vi "Online_SNR_Add_Measurement.vi"(8 "error in (no error)":errorcluster, 9 "Estimate":dbl format="%#_13g", 10 "True":dbl format="%#_13g", 11 "Online_SNR in":refnum<class "Online_SNR.lvclass">) -> (0 "error out":errorcluster, 3 "Online_SNR out":refnum<class "Online_SNR.lvclass">)   [LabVIEW 2021, in "Online_SNR.lvclass"]
uses:
  Online_SNR.lvclass
  Online_SNR.lvclass/Online_SNR.ctl
  Read Mean Square.vi
  Read Mean Square Error.vi
  Read N.vi
  Write Mean Square.vi
  Write Mean Square Error.vi
  Write N.vi
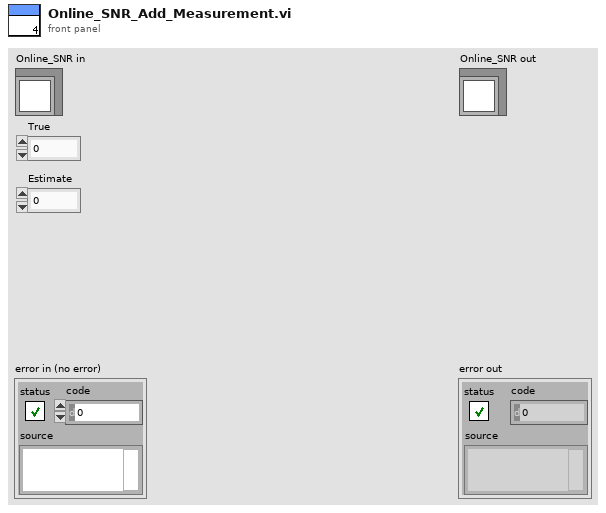
[diagram p1: front panel]
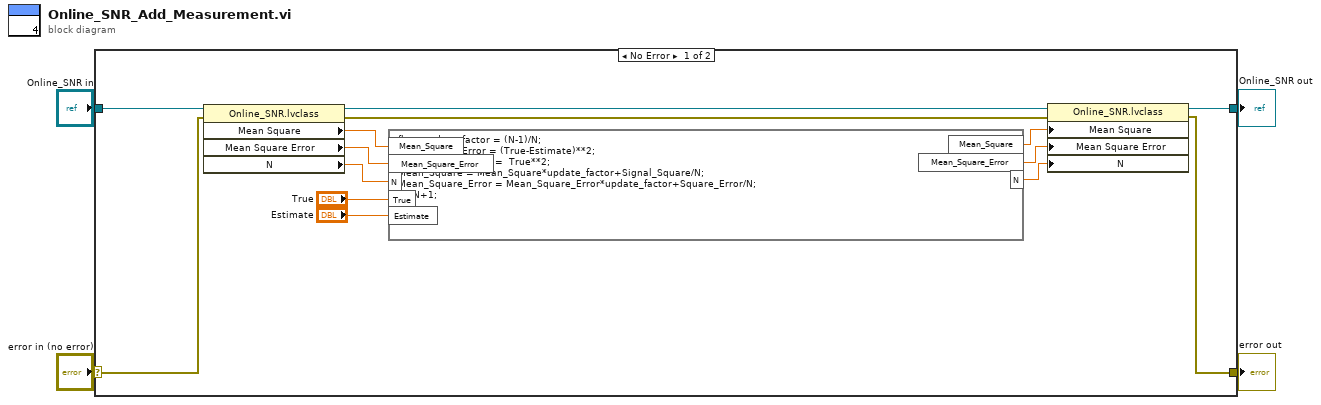
[diagram p0: block diagram]
diagram:
  n1 = case shown="No Error" "error in (no error)" {
    selector: "error in (no error)" -> [w6 w20]
    tunnel: [w5 w20] -> w3
    tunnel: [w9 w19] -> w1
    tunnel: "Online_SNR in" -> [w11 w19]
    frame No Error {
      n2 = property class="Online_SNR.lvclass"(reference=w11, error in=w6) -> (reference out=w10:refnum<class "Online_SNR.lvclass">, error out=w13:errorcluster, "Mean Square"=w18:dbl, "Mean Square Error"=w17:dbl, "N"=w16:dbl)
      n3 = formula code="float update_factor = (N-1)/N;\nfloat Square_Error = (True-Estimate)**2;\nfloat Signal_Square =  True**2;\nMean_Square = Mean_Square*update_factor+Signal_Square/N;\nMean_Square_Error = Mean_Square_Error*update_factor+Square_Error/N;\nN=N+1;"("Mean_Square"=w18, "Mean_Square_Error"=w17, "N"=w16, "True"="True", "Estimate"="Estimate") -> ("Mean_Square"=w8:dbl, "Mean_Square_Error"=w7:dbl, "N"=w12:dbl)
      n4 = property class="Online_SNR.lvclass"(reference=w10, error in=w13, "Mean Square"=w8, "Mean Square Error"=w7, "N"=w12) -> (reference out=w9:refnum<class "Online_SNR.lvclass">, error out=w5:errorcluster)
    }
    frame Error {
    }
  }
  "error out" <- w3
  "Online_SNR out" <- w1
